vi "subAcquisition_Waveform.vi"(6 "Waveform info":T3={"Waveform folder"=path "C:/Users/ZouOptics/Desktop/MATLAB codes/waveforms/12_waveforms.txt", "Movie frame rate (Hz)"=1000.0} {"Movie frame rate (Hz)" format="%0.0f"}, 7 "full path":path, 8 "error in (no error)":errorcluster, 10 "Waveform port selection":T2={"Dev2 DO lines"=["Dev2/port0/line3", "Dev2/port0/line5"], "Dev2 AO lines"=["Dev2/ao3", "Dev2/ao5"], "Patch AO line"="Dev1/ao0", "Dev1 AI lines"=["Dev1/ai0", "Dev1/ai8"], "Dev1 timing DO"="Dev1/port0/line1", "Camera timing DI"="Dev1/port0/line0", "Dev1 trigger source"="/Dev1/PFI0", "Dev2 trigger source"="/Dev2/PFI0"}, 11 "Handle in":u32) -> (0 "Error out":errorcluster, 2 "Acquisition params":T1={"Sampling rate (Hz)"=0.0, "dt (sec)"=0.0, "total time (sec)"=0.0, "# samples"=0, "Exposure time (ms)"=1000.0, "# frames"=0} {"Exposure time (ms)" format="%0.5f"; "Sampling rate (Hz)" format="%#.3f"}, 3 "Handle out":u32, 5 "AI Waveform":cluster{"xo":i32, dbl, "data":dbl[][]}(graph)={"xo"=0, 0.0001, "data"=array4x60000[240000 elements]})   [LabVIEW 2015]
panel:
  out "Camera info":cluster{"Handle in":u32, "Image file path":path}
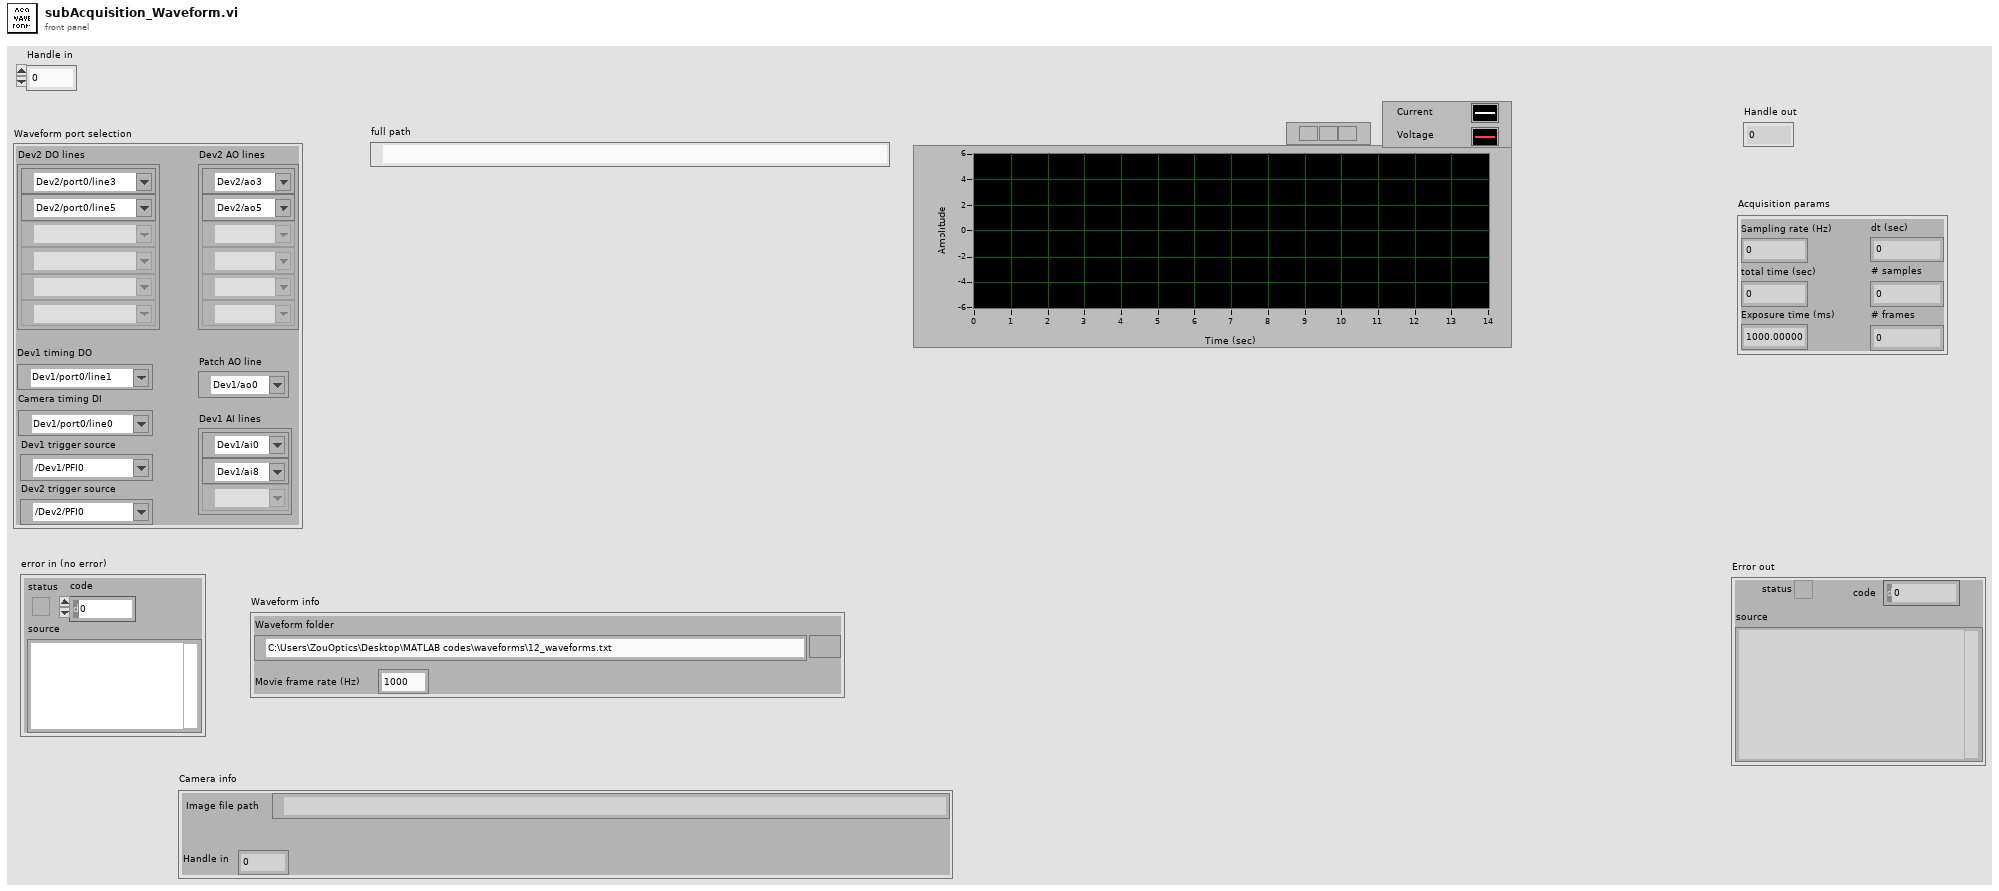
[diagram p1: front panel]
types:
  T1 = cluster{"Sampling rate (Hz)":dbl, "dt (sec)":dbl, "total time (sec)":dbl, "# samples":i32, "Exposure time (ms)":dbl, "# frames":i32}
  T2 = cluster{"Dev2 DO lines":tag[], "Dev2 AO lines":tag[], "Patch AO line":tag, "Dev1 AI lines":tag[], "Dev1 timing DO":tag, "Camera timing DI":tag, "Dev1 trigger source":tag, "Dev2 trigger source":tag}
  T3 = cluster{"Waveform folder":path, "Movie frame rate (Hz)":dbl}
  T4 = cluster{i32, "dt (sec)":dbl, "AI Waveform":dbl[][]}
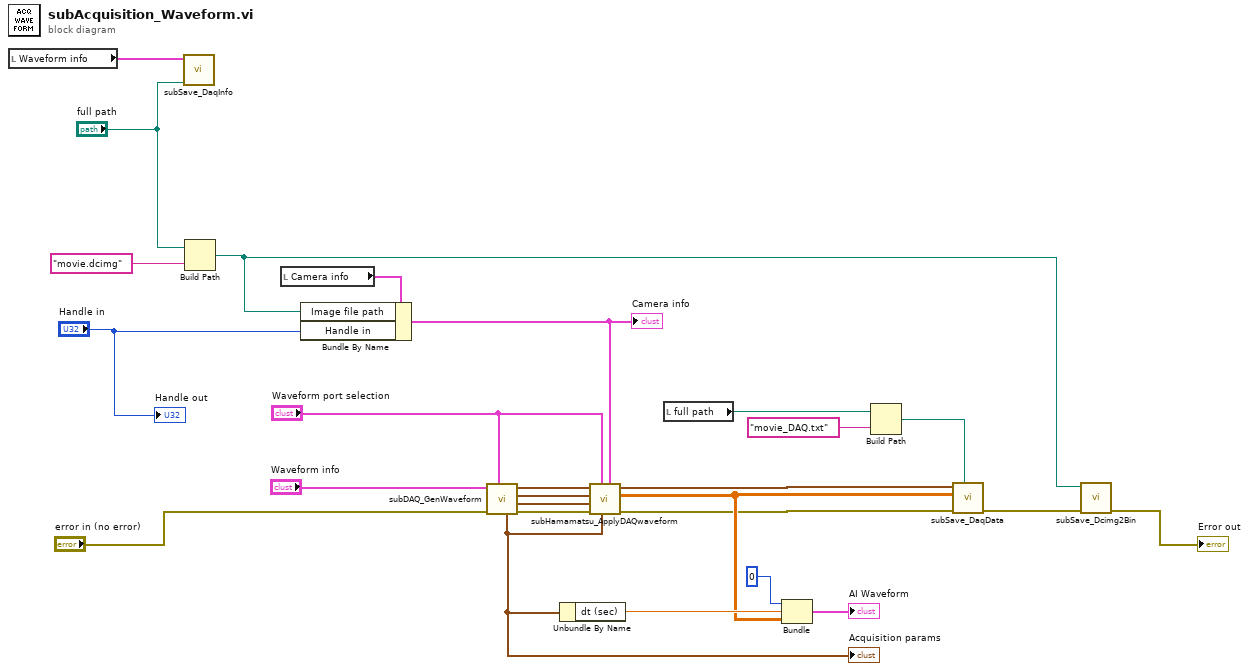
[diagram p0: block diagram]
diagram:
  n1 = local read "Waveform info"() -> (w8:T3)
  n2 = call "subSave_DaqInfo.vi"("full path"="full path", "Waveform info"=w8) -> ()  [unwired: 10 in]
  n3 = Build Path(base path="full path", name or relative path="movie.dcimg" ("Status")) -> (appended path=w19:path)
  n4 = local read "Camera info"() -> (w18:cluster{"Handle in":u32, "Image file path":path})
  n5 = Bundle By Name(cluster=w18, "Image file path"=w19, "Handle in"="Handle in") -> (w12:cluster{"Handle in":u32, "Image file path":path})
  "Camera info" <- w12
  n6 = call "subDAQ_GenWaveform.vi"("Waveform port selection"="Waveform port selection", "error in (no error)"="error in (no error)", "Waveform info"="Waveform info") -> ("error out"=w14:errorcluster, "Dev1 AO waveform"=w15:waveform(dbl), "Lasers AO waveform"=w16:waveform(dbl)[], "Lasers DO waveform"=w17:digitalwaveform[], "Acquisition params"=w11:T1)  [unwired: 4 in]
  "Acquisition params" <- w11
  n7 = Unbundle By Name(w11) -> ("dt (sec)"=w9:dbl)
  n8 = call "subHamamatsu_ApplyDAQwaveform.vi"("Camera info"=w12, "Acquisition params"=w11, "Waveform port selection"="Waveform port selection", "Camera in (no error)"=w14, "Dev1 AO waveform"=w15, "Dev2 AO waveform"=w16, "Dev2 DO waveform"=w17) -> ("Camera out"=w2:errorcluster, "AI Waveform"=w3:dbl[][], "Camera timging DI"=w4:digitalwaveform)  [unwired: 2 in]
  n9 = local read "full path"() -> (w6:path)
  n10 = Bundle(0, "dt (sec)"=w9, "AI Waveform"=w3) -> (→"AI Waveform":T4)  [unwired: 1 in]
  n11 = Build Path(base path=w6, name or relative path="movie_DAQ.txt") -> (appended path=w5:path)
  n12 = call "subSave_DaqData.vi"("path"=w5, "Camera in (no error)"=w2, "AI waveform"=w3, "DI waveform"=w4) -> ("Camera out"=w1:errorcluster)  [unwired: 7 in]
  n13 = call "subSave_Dcimg2Bin.vi"("Error in"=w1, ".dcimg file name"=w19) -> ("Error out"=→"Error out":errorcluster)  [unwired: 9 in]
  "Handle out" <- "Handle in"
